vi "Test Launch Root Actor Traces.vi"(8 "error in":errorcluster, 11 "Test Case In":refnum<class "Actor Trace Test.lvclass">) -> (0 "error out":errorcluster, 3 "Test Case Out":refnum<class "Actor Trace Test.lvclass">)   [LabVIEW 2020, in "Actor Trace.lvlib" / "Actor Trace Test.lvclass"]
uses:
  Actor Trace Test.lvclass
  C:/Program Files/National Instruments/LabVIEW 2024/vi.lib/Astemes/LUnit/Test Case.lvclass
  <vilib>/Astemes/LUnit/Test Case.lvclass/Test Case.ctl
  <vilib>/Astemes/LUnit/Append Pass Result.vi
  <vilib>/Astemes/LUnit/Run In UI.vi
  <vilib>/Utility/error.llb/Clear Errors.vi
  Core/ActorFramework/Actor/Actor.lvclass
  AF Trace Queue/AF Trace Queue.lvclass
  Core/ActorFramework/Stop Msg/Stop Msg.lvclass
  427b6f22-18f4-4bc5-a6f5-1b704fac43be.vi
  <vilib>/Astemes/LUnit/Test Case.lvclass
panel:
  out "Trace Data":string[](array[string])
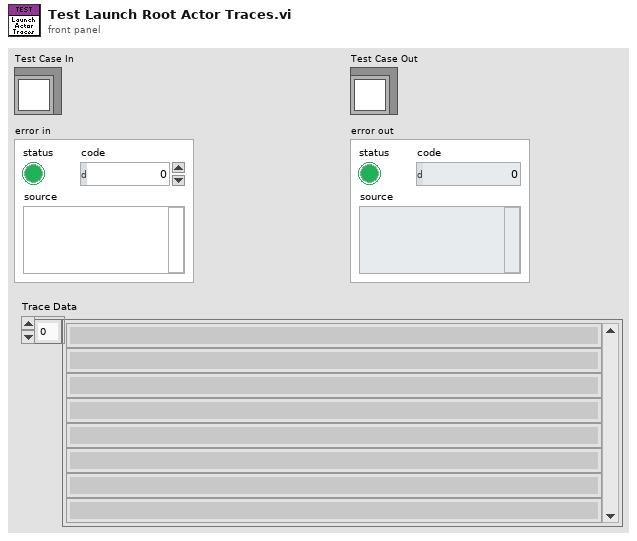
[diagram p1: front panel]
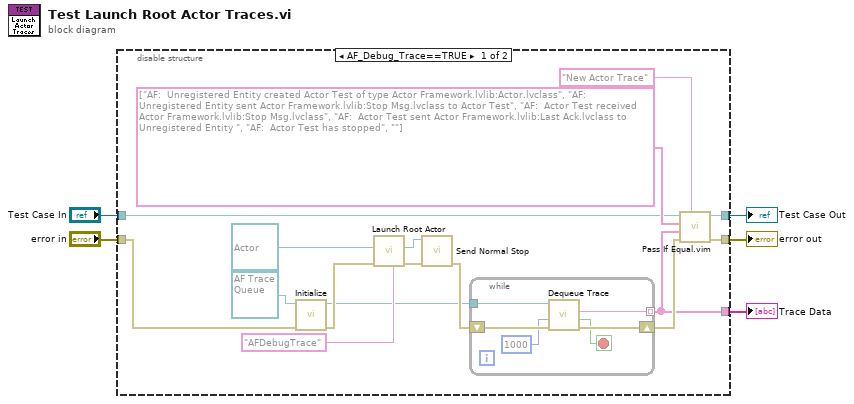
[diagram p0: block diagram]
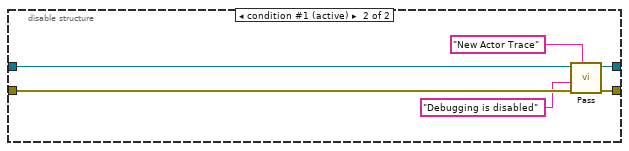
[diagram p2: hidden frame]
diagram:
  n1 = disable-structure shown="AF_Debug_Trace==TRUE" {
    disable-tunnel: "error in" -> [w18 w33]
    disable-tunnel: [w16 w32] -> w4
    disable-tunnel: [w9 _] -> w3
    disable-tunnel: [w8 w30] -> w2
    disable-tunnel: "Test Case In" -> [w7 w29]
    frame condition #0 {
      n2 = call-dynamic "Initialize.vi"("error in"=w18, "AF Trace Queue in"=refnum<class "AF Trace Queue.lvclass"> refnum) -> ("error out"=w21:errorcluster, "AF Trace Queue out"=w6:refnum<class "AF Trace Queue.lvclass">)  [unwired: 8 in]
      n3 = call "Launch Root Actor.vi"("Debug Alias"="AFDebugTrace", "error in (no error)"=w21, "Actor"=refnum<class "Actor.lvclass"> refnum ("Actor Framework:Actor")) -> ("error out"=w20:errorcluster, "Actor's Enqueuer"=w14:refnum<class "Message Enqueuer.lvclass">)  [unwired: 7 in]
      n4 = call "Send Normal Stop.vi"("error in (no error)"=w20, "Message Enqueuer"=w14) -> ("error out"=w19:errorcluster)  [unwired: 9 in]
      n5 = while {
        tunnel: w6 -> [w25]
        shift-right: [w26] -> w17
        shift-left: w19 -> [w27]
        tunnel: [w22] -> w9 mode=indexing
        stop <- w23 stop-if-true
        n6 = call "Dequeue Trace.vi"("error in (no error)"=w27, "timeout in ms (-1)"=1000, "AF Trace Queue in"=w25) -> ("error out"=w26:errorcluster, "timed out?"=w23:bool, "Trace String"=w22:string)  [unwired: 5 in, 1 out]
      }
      n7 = call "Pass If Equal.vim"("Description"="New Actor Trace" ("Label (VI Title)"), "error in (no error)"=w17, "Actual"=w9, "Expected"=string[] ["AF:  Unregistered Entity created Actor Test of type Actor Framework.lvlib:Actor.lvclass", "AF:  Unregistered Entity sent Actor Framework.lvlib:Stop Msg.lvclass to Actor Test", "AF:  Actor Test received Actor Framework.lvlib:Stop Msg.lvclass", "AF:  Actor Test sent Actor Framework.lvlib:Last Ack.lvclass to Unregistered Entity ", "AF:  Actor Test has stopped", ""] ("Array"), "LUnit Test Case In"=w7) -> ("error out"=w16:errorcluster, "LUnit Test Case Out"=w8:refnum<class "Actor Trace Test.lvclass">)  [unwired: 5 in]
    }
    frame condition #1 (active) {
      n8 = call <vilib>:"Pass.vi"("Description"="New Actor Trace" ("Label (VI Title)"), "error in (no error)"=w33, "Message"="Debugging is disabled", "LUnit Test Case In"=w29) -> ("error out"=w32:errorcluster, "LUnit Test Case Out"=w30:refnum<class "Actor Trace Test.lvclass">)  [unwired: 6 in]
    }
  }
  "Trace Data" <- w3
  "Test Case Out" <- w2
  "error out" <- w4
